vi "Reserve Device for Function.vi"(8 "error in (no error)":errorcluster, 10 "Device (GUID) to Reserve":string, 11 "Controller in":refnum<class "Controller.lvclass">) -> (0 "error out":errorcluster, 3 "Controller out":refnum<class "Controller.lvclass">)   [LabVIEW 2016, in "Controller Actor.lvlib" / "Controller.lvclass"]
uses:
  <userlib>/Common Components/Controller/Controller.lvclass
  <userlib>/Common Components/Controller UI/Update DT event data.ctl
  <userlib>/Common Components/Controller UI/Update DT Cmd.ctl
  <userlib>/Common Components/Controller UI/Update DT event data - checked out.ctl
  <userlib>/Common Components/Controller UI Messages/Update DT Event Msg/Update DT Event Msg.lvclass/Update DT Event Msg.ctl
  <vilib>/ActorFramework/Message Enqueuer/Message Enqueuer.lvclass/Message Enqueuer.ctl
  <vilib>/ActorFramework/Message Enqueuer/Enqueue.vi
  <userlib>/Common Components/Controller UI Messages/Update DT Event Msg/Update DT Event Msg.lvclass
  C:/Program Files (x86)/National Instruments/LabVIEW 2016/vi.lib/ActorFramework/Message/Message.lvclass
  <vilib>/ActorFramework/Message Priority Queue/Priority Enqueue.vi
  <userlib>/Common Components/Controller UI/Controller UI.lvclass
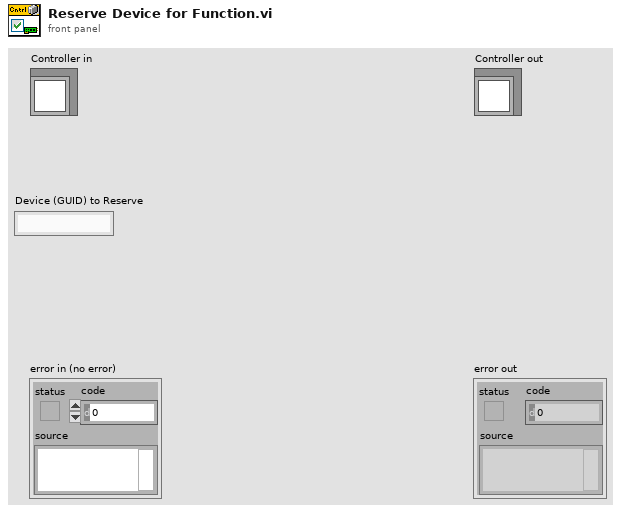
[diagram p1: front panel]
types:
  T1 = typedef "Controller UI.lvlib/Controller UI.lvclass/Update DT event data - checked out.ctl" = cluster{"GUID":string, "checked-out?":bool}
  T2 = typedef "Controller UI.lvlib/Controller UI.lvclass/Update DT event data.ctl" = cluster{"Cmd":T3, "Data Array":variant[]}
  T3 = typedef "Controller UI.lvlib/Controller UI.lvclass/Update DT Cmd.ctl" = enum16{"Update HWtype\\HWplugin array", "Update Checked-out", "Update COMM Status", "Load DevInfo from File", "Save DevInfo to File", "Update COMM Address List"}
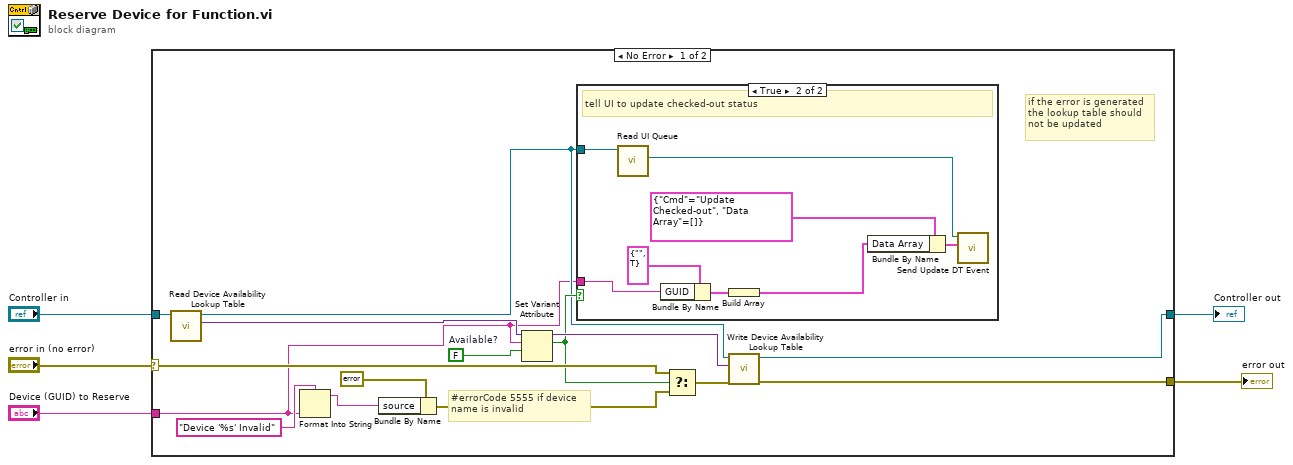
[diagram p0: block diagram]
diagram:
  n1 = case shown="No Error" "error in (no error)" {
    selector: "error in (no error)" -> [w12 w30]
    tunnel: [w10 w30] -> w4
    tunnel: [w17 w29] -> w2
    tunnel: "Controller in" -> [w19 w29]
    tunnel: "Device (GUID) to Reserve" -> [w7 _]
    frame No Error {
      w6 = FALSE  # Available?
      # "if the error is generated\nthe lookup table should\nnot be updated"
      # "#errorCode 5555 if device\nname is invalid"
      n2 = call <userlib>:"Read Device Availability Lookup Table.vi"("Controller in"=w19) -> ("Device Availability Lookup Table"=w20:variant, "Controller out"=w8:refnum<class "Controller.lvclass">)  [unwired: 8 in, 1 out]
      n3 = Format Into String(format string="Device '%s' Invalid" ("source"), w7) -> (resulting string=w15:string)  [unwired: 2 in, 1 out]
      n4 = Bundle By Name(cluster=errorcluster {"status"=TRUE, "code"=5555, "source"="Device '%s' Invalid"} ("error constant"), "source"=w15) -> (w13:errorcluster)
      n5 = Set Variant Attribute(Variant=w20, name=w7, value=w6) -> (Variant out=w18:variant, replaced=w9:bool)  [unwired: 1 in, 1 out]
      n6 = case shown="True" w9 {
        tunnel: w8 -> [_ w28]
        tunnel: w7 -> [_ w24]
        frame False {
        }
        frame True {
          # "tell UI to update checked-out status"
          n7 = call <userlib>:"Read UI Queue.vi"("UI Controller in"=w28) -> ("UI Queue"=w27:refnum<class "Message Enqueuer.lvclass">)  [unwired: 8 in, 2 out]
          n8 = Bundle By Name(cluster=T1 {"GUID"="", "checked-out?"=TRUE} ("Cluster"), "GUID"=w24) -> (w23:T1)
          n9 = Build Array(w23) -> (w22:T1[])
          n10 = Bundle By Name(cluster=T2 {"Cmd"=enum."Update Checked-out", "Data Array"=[]} ("event data"), "Data Array"=w22) -> (w25:T2)
          n11 = call <userlib>:"Send Update DT Event.vi"("event data"=w25, "Message Enqueuer"=w27) -> ()  [unwired: 8 in, 2 out]
        }
      }
      n12 = Select(t=w12, s=w9, f=w13) -> (s? t:f=w11:errorcluster)
      n13 = call <userlib>:"Write Device Availability Lookup Table.vi"("error in (no error)"=w11, "Device Availability Lookup Table"=w18, "Controller in"=w8) -> ("error out"=w10:errorcluster, "Controller out"=w17:refnum<class "Controller.lvclass">)  [unwired: 7 in]
    }
    frame Error {
    }
  }
  "error out" <- w4
  "Controller out" <- w2
